vi "Linear fit test.vi"   [LabVIEW 2009]
uses:
  <vilib>/Analysis/NI_AALPro.lvlib
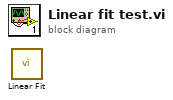
[diagram p0: block diagram]
diagram:
  n1 = call <vilib>:"Linear Fit.vi"() -> ()  [unwired: 11 in, 5 out]
